vi "TIO Device Close.vi"(8 "Error in":errorcluster, 11 "TIO":T1={"TC Connection"={"Type"=enum."Serial", "URL"="serial:///dev/cu.usbserial-00000", "TO"=500, "Addr"=0, "Port"=0, "TCP"=refnum, "UDP"=refnum, "Route"=""}, "REQ"=refnum, "REP"=refnum}) -> ()   [LabVIEW 2010]
panel:
  # "TIO Tick"
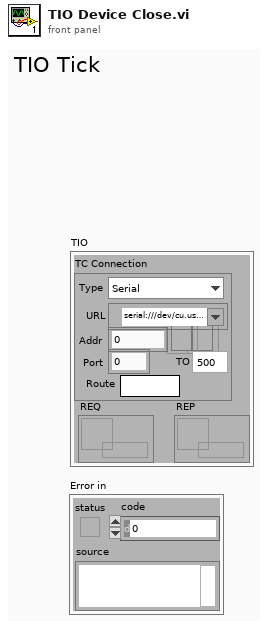
[diagram p1: front panel]
types:
  T1 = cluster{"TC Connection":cluster{"Type":enum16{"Serial", "TCP", "UDP", "mUDP"}, "URL":refnum<visa-resource-name>, "TO":u32, "Addr":u32, "Port":i32, "TCP":refnum<k5>, "UDP":refnum<k16>, "Route":string}, "REQ":refnum<queue>, "REP":refnum<queue>}
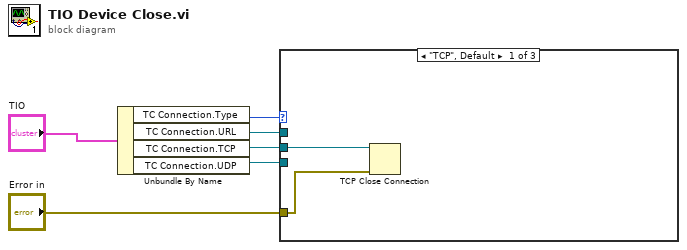
[diagram p0: block diagram]
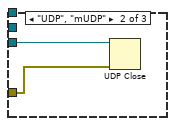
[diagram p2: hidden frame]
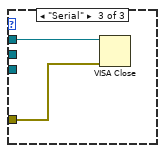
[diagram p3: hidden frame]
diagram:
  n1 = Unbundle By Name("TIO") -> ("TC Connection.Type"=w5:enum16{"Serial", "TCP", "UDP", "mUDP"}, "TC Connection.URL"=w4:refnum<visa-resource-name>, "TC Connection.TCP"=w2:refnum<k5>, "TC Connection.UDP"=w1:refnum<k16>)
  n2 = case shown="\"TCP\", Default" w5 {
    tunnel: w4 -> [_ _ w12]
    tunnel: "Error in" -> [w7 w10 w11]
    tunnel: w2 -> [w8 _ _]
    tunnel: w1 -> [_ w9 _]
    frame "TCP", Default {
      n3 = TCP Close Connection(connection ID=w8, error in (no error)=w7) -> ()  [unwired: 1 in, 2 out]
    }
    frame "UDP", "mUDP" {
      n4 = UDP Close(connection ID=w9, 8:w10) -> ()  [unwired: 2 out]
    }
    frame "Serial" {
      n5 = VISA Close(VISA resource name=w12, error in (no error)=w11) -> ()  [unwired: 1 out]
    }
  }
